vi "Call Version Message.vi"(0 "VISA resource name out":refnum<visa-resource-name>, 1 "delay before read (ms)":u32=500, 5 "error in":errorcluster) -> (4 "bytes read":u32=33, 6 "read string":string="Ver. 0.1, Feb 10 2013, 23:27:07\r\n", 7 "VISA Out":refnum<visa-resource-name>, 8 "error out":errorcluster)   [LabVIEW 2012]
doc: "The Basic Serial Read and Write example performs a Serial Port Read, a Serial Port Write, or a combination of these actions. The user selects the actions (read or write) on the front panel. If both are selected, the VI will write the data first, read data, and then close the VISA session that is opened to the port. This VI will wait until the specified number of bytes is received at the port or until a termination character is read.\n\nINSTRUCTIONS:\n1) Select the serial resource and configuration parameters (baud rate, data bits, parity, stop bits, flow control).\n2) Select the operations to be performed. \n3) Connect the serial port to your device. If no device is available, perform a loopback test by doing one of the following. Short pins 2 and 3 on a RS-232 cable or short pin 4 to pin 8 and pin 5 to pin 9 on a RS-485/422 cable. \n4) Run the VI to see the data read. (The \"read string\" will match the \"string to write\" if a loopback test was performed.)\n\nNote: The parameters set for the serial port must match the parameters of the connected instrument or device. In this example, the bytes to read parameter specifies the number of bytes that the serial port reads. If there were more bytes at the port than the number specified in bytes to read, those bytes would not be read. Also, if you specify to read more bytes than the number of bytes actually read, you might receive a timeout error message.\n\nOn the block diagram, the Configure Serial Port VI sets the configuration parameters. The front panel displays the controls used to configure the basic parameters, such as baud rate, data bits, and parity. Constants configure the other parameters the user probably does not need set. After the VISA Configure Serial Port VI opens the VISA session and configures the port, the VI passes the VISA resource name to other VIs that perform operations on that VISA resource. The VISA Write function sends a command to the serial device and the VISA Read function returns data based on the command. The VISA Close function then closes the reference to the serial device. It is important to close the reference; otherwise communication through with that port through protocols other than VISA might not be possible."
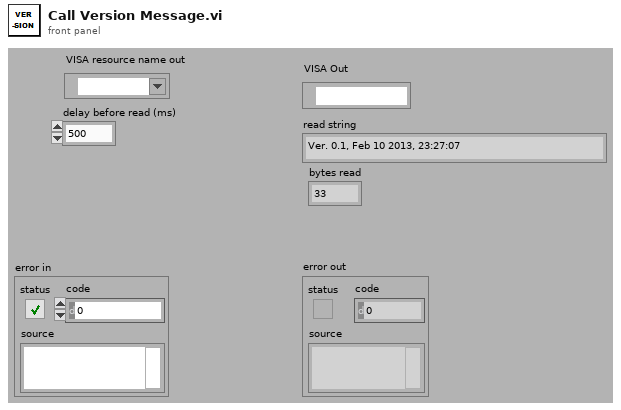
[diagram p1: front panel]
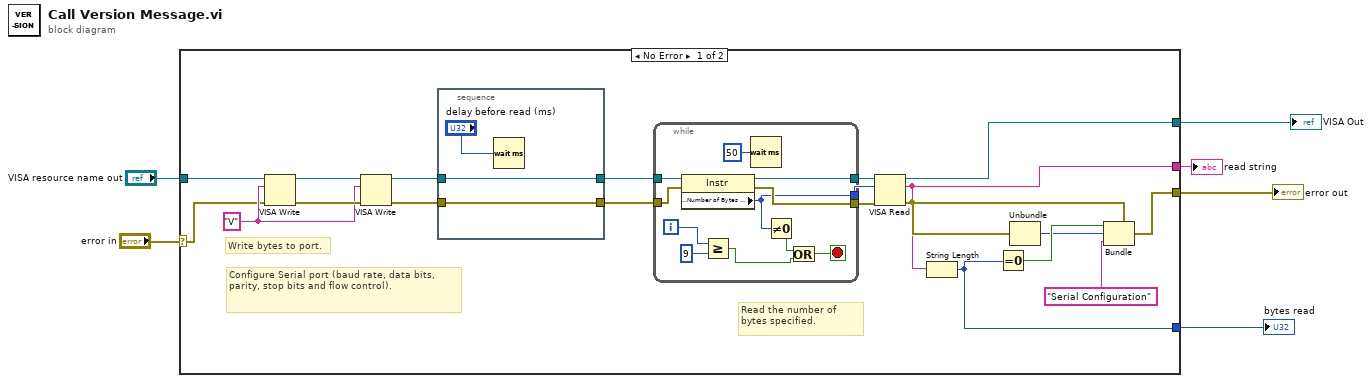
[diagram p0: block diagram]
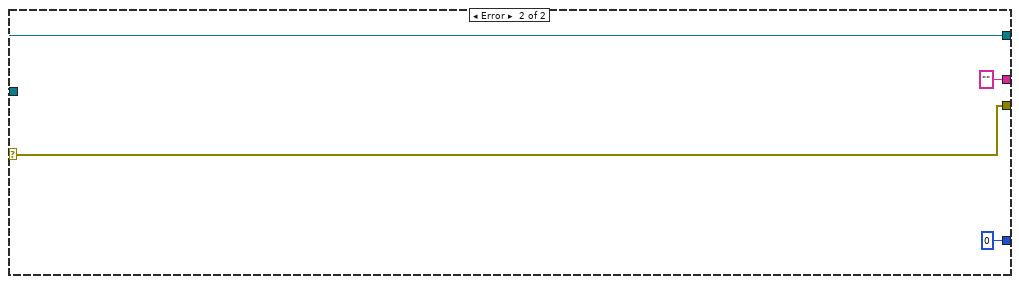
[diagram p2: hidden frame]
diagram:
  n1 = case shown="No Error" "error in" {
    selector: "error in" -> [w7 w44]
    tunnel: [w26 w43] -> w6
    tunnel: "VISA resource name out" -> [w16 w43]
    tunnel: [w20 w44] -> w4
    tunnel: [w9 0] -> w2
    tunnel: [w8 "" ("read buffer")] -> w1
    frame No Error {
      w12 = "V" ("string to write")
      # "Read the number of bytes specified."
      # "Write bytes to port."
      # "Configure Serial port (baud rate, data bits, parity, stop bits and flow control)."
      n2 = VISA Write(VISA resource name=w16, write buffer=w12, error in (no error)=w7) -> (VISA resource name out=w14:refnum<visa-resource-name>, error out=w13:errorcluster)  [unwired: 1 out]
      n3 = VISA Write(VISA resource name=w14, write buffer=w12, error in (no error)=w13) -> (VISA resource name out=w11:refnum<visa-resource-name>, error out=w10:errorcluster)  [unwired: 1 out]
      n4 = stacked-sequence {
        tunnel: w10 -> [w40]
        tunnel: [w40] -> w25
        tunnel: w11 -> [w39]
        tunnel: [w39] -> w24
        frame #0 {
          n5 = Wait (ms)(milliseconds to wait="delay before read (ms)") -> ()  [unwired: 1 out]
        }
      }
      n6 = while {
        tunnel: w25 -> [w37]
        tunnel: w24 -> [w36]
        tunnel: [w35] -> w23
        tunnel: [w34] -> w22
        tunnel: [w28] -> w15
        i -> [w30]
        stop <- w31 stop-if-true
        n7 = property class="Instr"(reference=w36, error in=w37) -> (reference out=w35:refnum<visa-resource-name>, error out=w34:errorcluster, "Serial Settings:Number of Bytes at Serial Port"=w28:u32)
        n8 = Greater Or Equal?(x=w30, y=9) -> (x >= y?=w27:bool)
        n9 = Wait (ms)(milliseconds to wait=u32 50) -> ()  [unwired: 1 out]
        n10 = Not Equal To 0?(x=w28) -> (x != 0?=w32:bool)
        n11 = Or(x=w32, y=w27) -> (x .or. y?=w31:bool)
      }
      n12 = VISA Read(VISA resource name=w23, byte count=w15, error in (no error)=w22) -> (VISA resource name out=w26:refnum<visa-resource-name>, read buffer=w8:string, error out=w21:errorcluster)  [unwired: 1 out]
      n13 = String Length(string=w8) -> (length=w9:i32)
      n14 = Equal To 0?(x=w9) -> (x = 0?=w19:bool)
      n15 = Unbundle(w21) -> ("code"=w17:i32)  [unwired: 2 out]
      n16 = Bundle(cluster=w21, "status"=w19, "code"=w17, "source"="Serial Configuration") -> (w20:errorcluster)
    }
    frame Error {
    }
  }
  "error out" <- w4
  "VISA Out" <- w6
  "bytes read" <- w2
  "read string" <- w1
